vi "M1 Titanium Metal Properties.vi"(6 "m-nm M1":dbl, 9 "Metal 1 (Ti)":dbl, 10 "Energy (Heat; I^2R)":dbl, 11 "NS Base Area":dbl) -> (1 "Volume M1":dbl, 2 "Mass M1":dbl, 3 "Delta Temp Change M1":dbl, 4 "M1 Thickness":dbl, 5 "M1 Specfic Heat Capacity":dbl, 7 "M1 Density":dbl, 8 "mc":dbl)   [LabVIEW 2020]
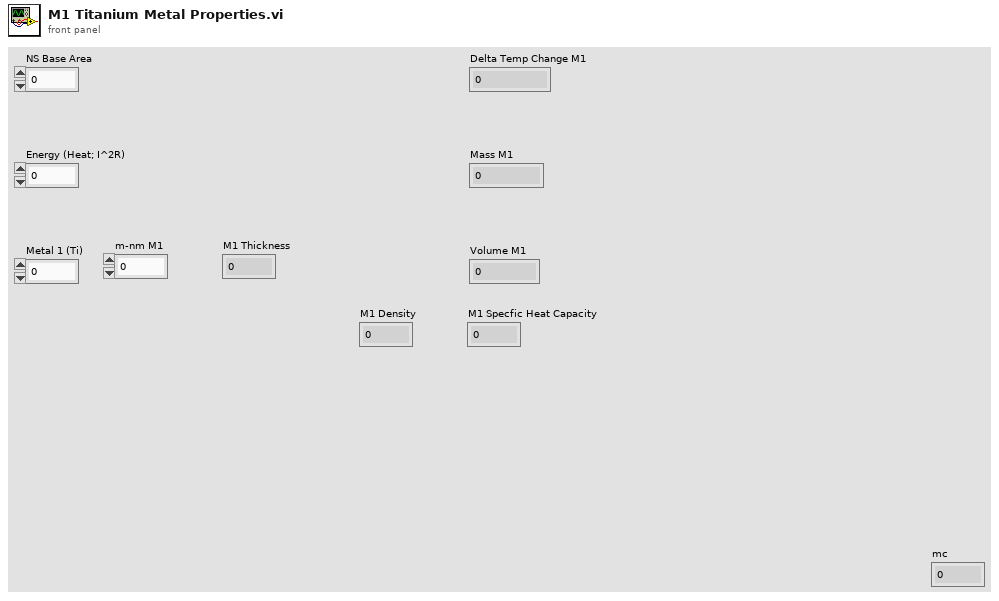
[diagram p1: front panel]
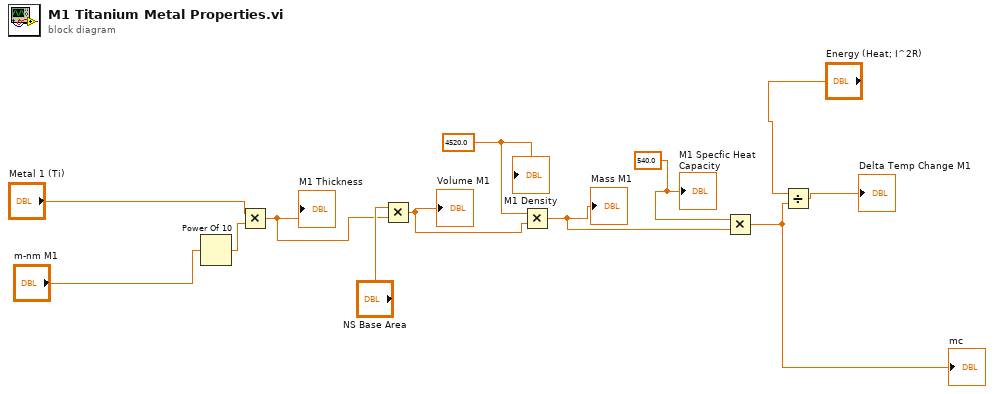
[diagram p0: block diagram]
diagram:
  w10 = 540.0 ("Silicon Specfic Heat Capacity 3")
  w6 = 4520.0 ("Silicon Density 3")
  n1 = Power Of 10(x="m-nm M1") -> (10^x=w2:dbl)
  n2 = Multiply(x="Metal 1 (Ti)", y=w2) -> (x*y=w5:dbl)
  "M1 Thickness" <- w5
  n3 = Multiply(x="NS Base Area", y=w5) -> (x*y=w7:dbl)
  "Volume M1" <- w7
  n4 = Multiply(x=w6, y=w7) -> (x*y=w9:dbl)
  "Mass M1" <- w9
  n5 = Multiply(x=w10, y=w9) -> (x*y=w1:dbl)
  "mc" <- w1
  n6 = Divide(x="Energy (Heat; I^2R)", y=w1) -> (x/y=→"Delta Temp Change M1":dbl)
  "M1 Density" <- w6
  "M1 Specfic Heat Capacity" <- w10
